vi "MGCC_StaEst_opal_RT_convertPnode.vi"(10 "cluster":T1) -> (0 "error out 2":errorcluster, 1 "error out 3":errorcluster, 2 "P_node":T1)   [LabVIEW 2016]
uses:
  Model Management/Global_MdlMgmt.vi
  <vilib>/Utility/error.llb/Error Cluster From Error Code.vi
  MGCC_StaEst_global.vi
  Finite State Machine/Sub-VIs/MGCC_FntStaMach_gobal.vi
  <vilib>/imath/engines/lvmath2/RunTimeEngine/IndexRead/NIMS M($,S).vi
  <instcachedir>/0/NIMS M($,S)_3E5749BBB62E49528D4765A77F1F6D98.lvgen/NIMS M($,S)_3E5749BBB62E49528D4765A77F1F6D98_001.vi
  <vilib>/imath/engines/lvmath2/RunTimeEngine/BuiltInFunctions/length/NIMS_length(GV).vi
  <instcachedir>/0/NIMS_length(GV)_08A3D13377FD4E4B96F5795FBF3698FA.lvgen/NIMS_length(GV)_08A3D13377FD4E4B96F5795FBF3698FA_001.vi
  <vilib>/imathl/engines/lvmath/Functions/Error Handling/Create Error.vi
  <vilib>/imath/engines/lvmath2/RunTimeEngine/RangeToken/NIMS_Range_R3 - Integer.vi
  <instcachedir>/0/NIMS_Range_R3 - Integer_A435E2FF893B4C718FD5055FE39FE2F6.lvgen/NIMS_Range_R3 - Integer_A435E2FF893B4C718FD5055FE39FE2F6_000.vi
  <vilib>/imath/engines/lvmath2/RunTimeEngine/CommandStatement/MC_CommandStatement_break.vi
  <vilib>/imath/engines/lvmath2/RunTimeEngine/IndexRead/NIMS V(S).vi
  <instcachedir>/0/NIMS V(S)_0488751826AF41519A22953C041130DC.lvgen/NIMS V(S)_0488751826AF41519A22953C041130DC_000.vi
  <vilib>/imath/engines/lvmath2/RunTimeEngine/IndexReplace/NIMS M(S,$)=V.vi
  <instcachedir>/0/NIMS M(S,$)=V_BCCFA522A894489B8FA760383D74A164.lvgen/NIMS M(S,$)=V_BCCFA522A894489B8FA760383D74A164_001.vi
  <instcachedir>/0/NIMS M($,S)_3E5749BBB62E49528D4765A77F1F6D98.lvgen/NIMS M($,S)_3E5749BBB62E49528D4765A77F1F6D98_000.vi
  <instcachedir>/0/NIMS_length(GV)_08A3D13377FD4E4B96F5795FBF3698FA.lvgen/NIMS_length(GV)_08A3D13377FD4E4B96F5795FBF3698FA_000.vi
  <vilib>/imath/engines/lvmath2/RunTimeEngine/IndexRead/NIMS M(S,S).vi
  <instcachedir>/0/NIMS M(S,S)_AC51E74150A542F7991B9634C66F3096.lvgen/NIMS M(S,S)_AC51E74150A542F7991B9634C66F3096_000.vi
  <vilib>/imath/engines/lvmath2/RunTimeSupport/NIMS_Error if Not Equal.vi
  <instcachedir>/0/NIMS_Error if Not Equal_43252A79AD05436189442EC0C5E5AB8A.lvgen/NIMS_Error if Not Equal_43252A79AD05436189442EC0C5E5AB8A_000.vi
  <vilib>/imath/engines/lvmath2/RunTimeEngine/ErrorHandling/NIMS_Create Error From Enums.vi
  <vilib>/imath/engines/lvmath2/RunTimeEngine/IndexRead/NIMS M(S,$).vi
  <instcachedir>/0/NIMS M(S,$)_F24F360562DE41D8BE234322A2E15C65.lvgen/NIMS M(S,$)_F24F360562DE41D8BE234322A2E15C65_001.vi
  <vilib>/imath/engines/lvmath2/RunTimeEngine/NodeEndStatement/NIMS_NodeEndStatement_Output.vi
  <instcachedir>/0/NIMS_NodeEndStatement_Output_53EC0D466D134D7ABD903AC30B43404B.lvgen/NIMS_NodeEndStatement_Output_53EC0D466D134D7ABD903AC30B43404B_003.vi
  <vilib>/imath/engines/lvmath2/RunTimeEngine/ErrorHandling/NIMS_Finalize Error.vi
  <vilib>/ErrorRing/Error Ring.xnode
panel:
  out "array w/ subset deleted":dbl[](array[numeric])
  out "f_MGCC_OnliTopoIden_EnergizedMatrix 2":dbl[](array[numeric])
  out "State_est BESS location":dbl[](array[numeric])
  out "Slack_bus":dbl[](array[numeric])
  out "element":dbl
  out "f_MGCC_OnliTopoIden_EnergizedMatrix":dbl[](array[numeric])
  out "error out":errorcluster
  out "p_node 2":cdb[][](array[numeric])
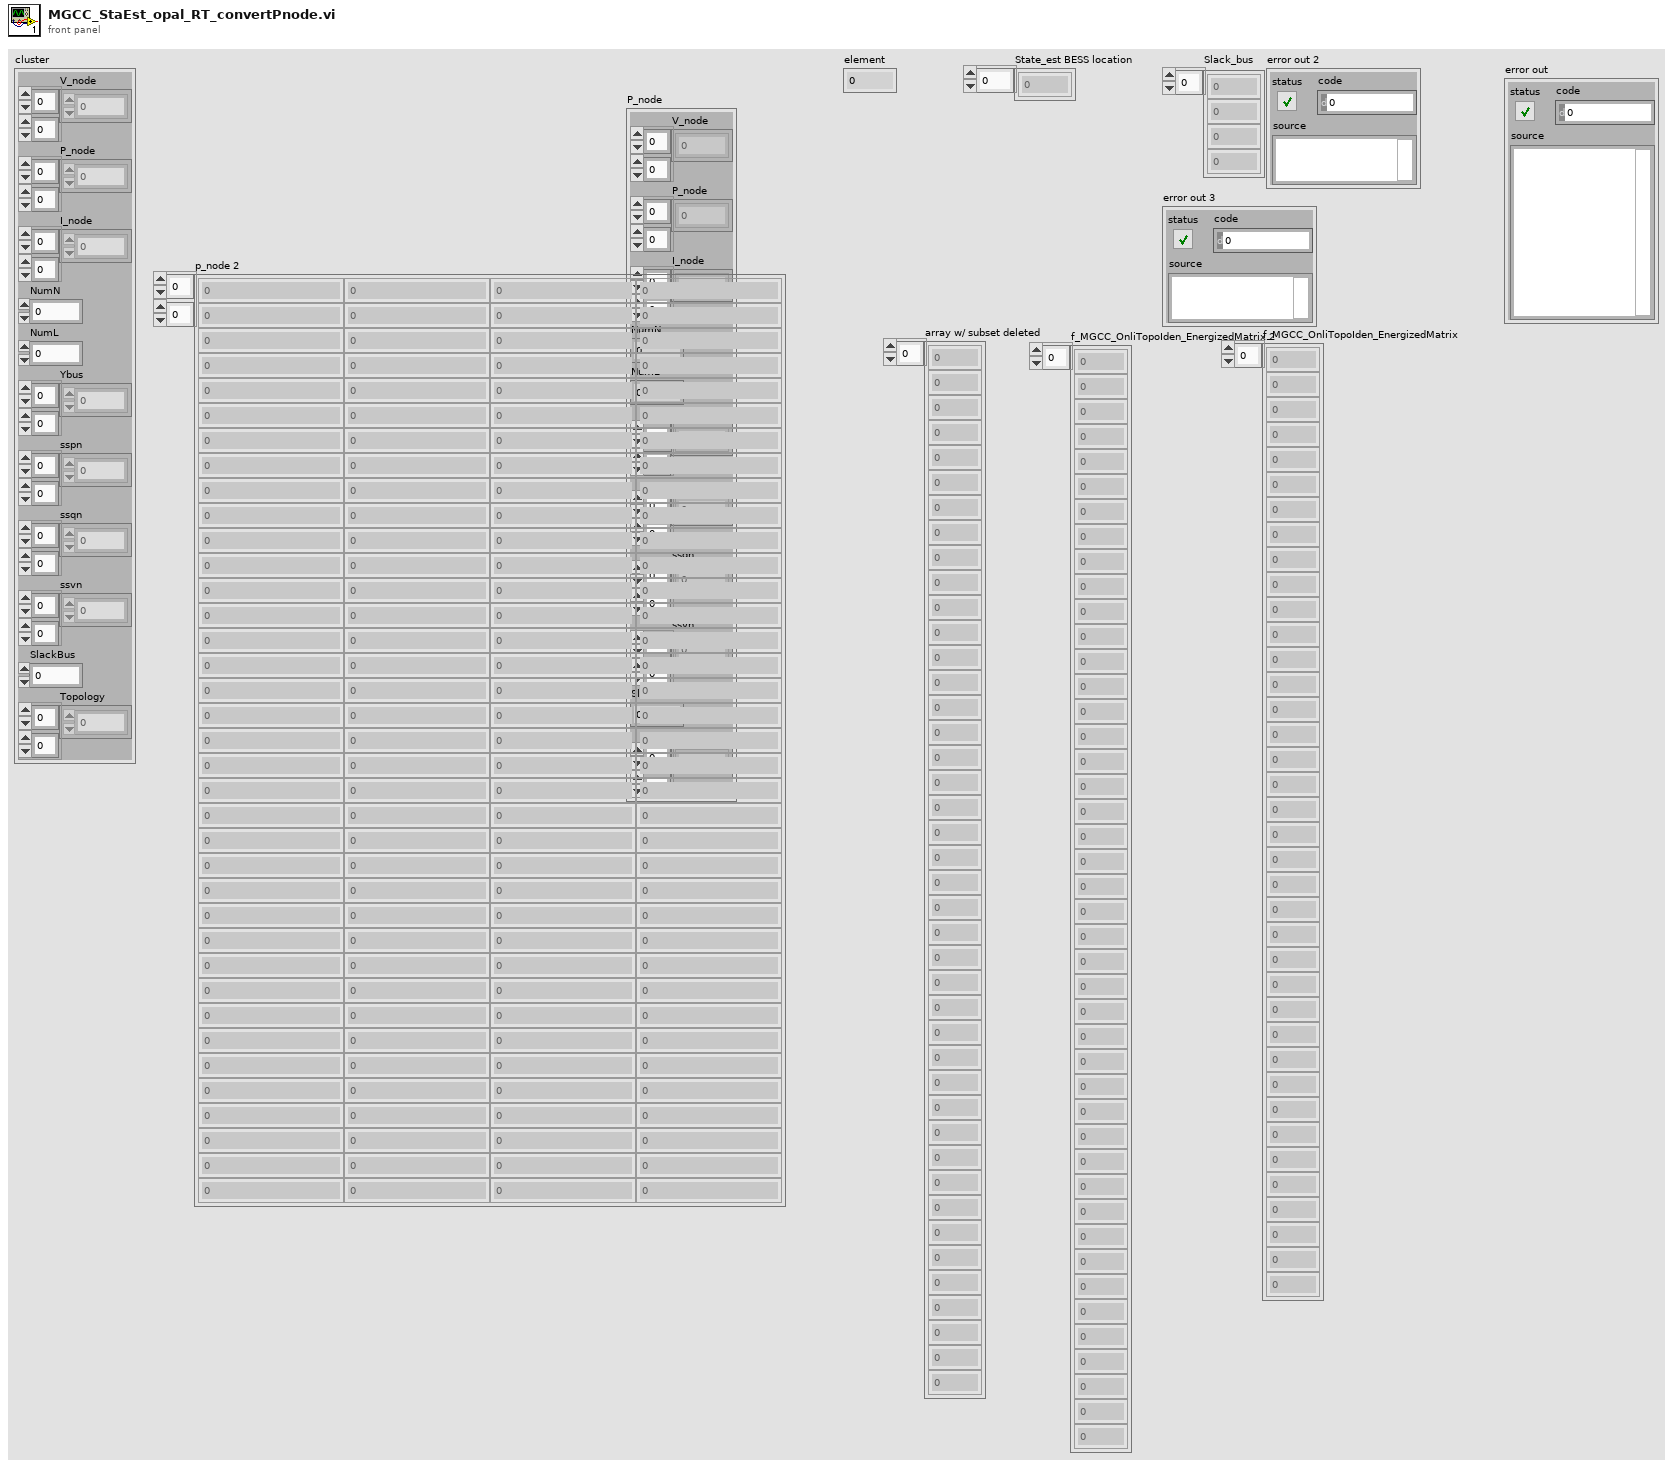
[diagram p1: front panel]
types:
  T1 = cluster{"V_node":cdb[][], "P_node":cdb[][], "I_node":cdb[][], "NumN":dbl, "NumL":dbl, "Ybus":cdb[][], "sspn":dbl[][], "ssqn":dbl[][], "ssvn":dbl[][], "SlackBus":dbl, "Topology":dbl[][]}
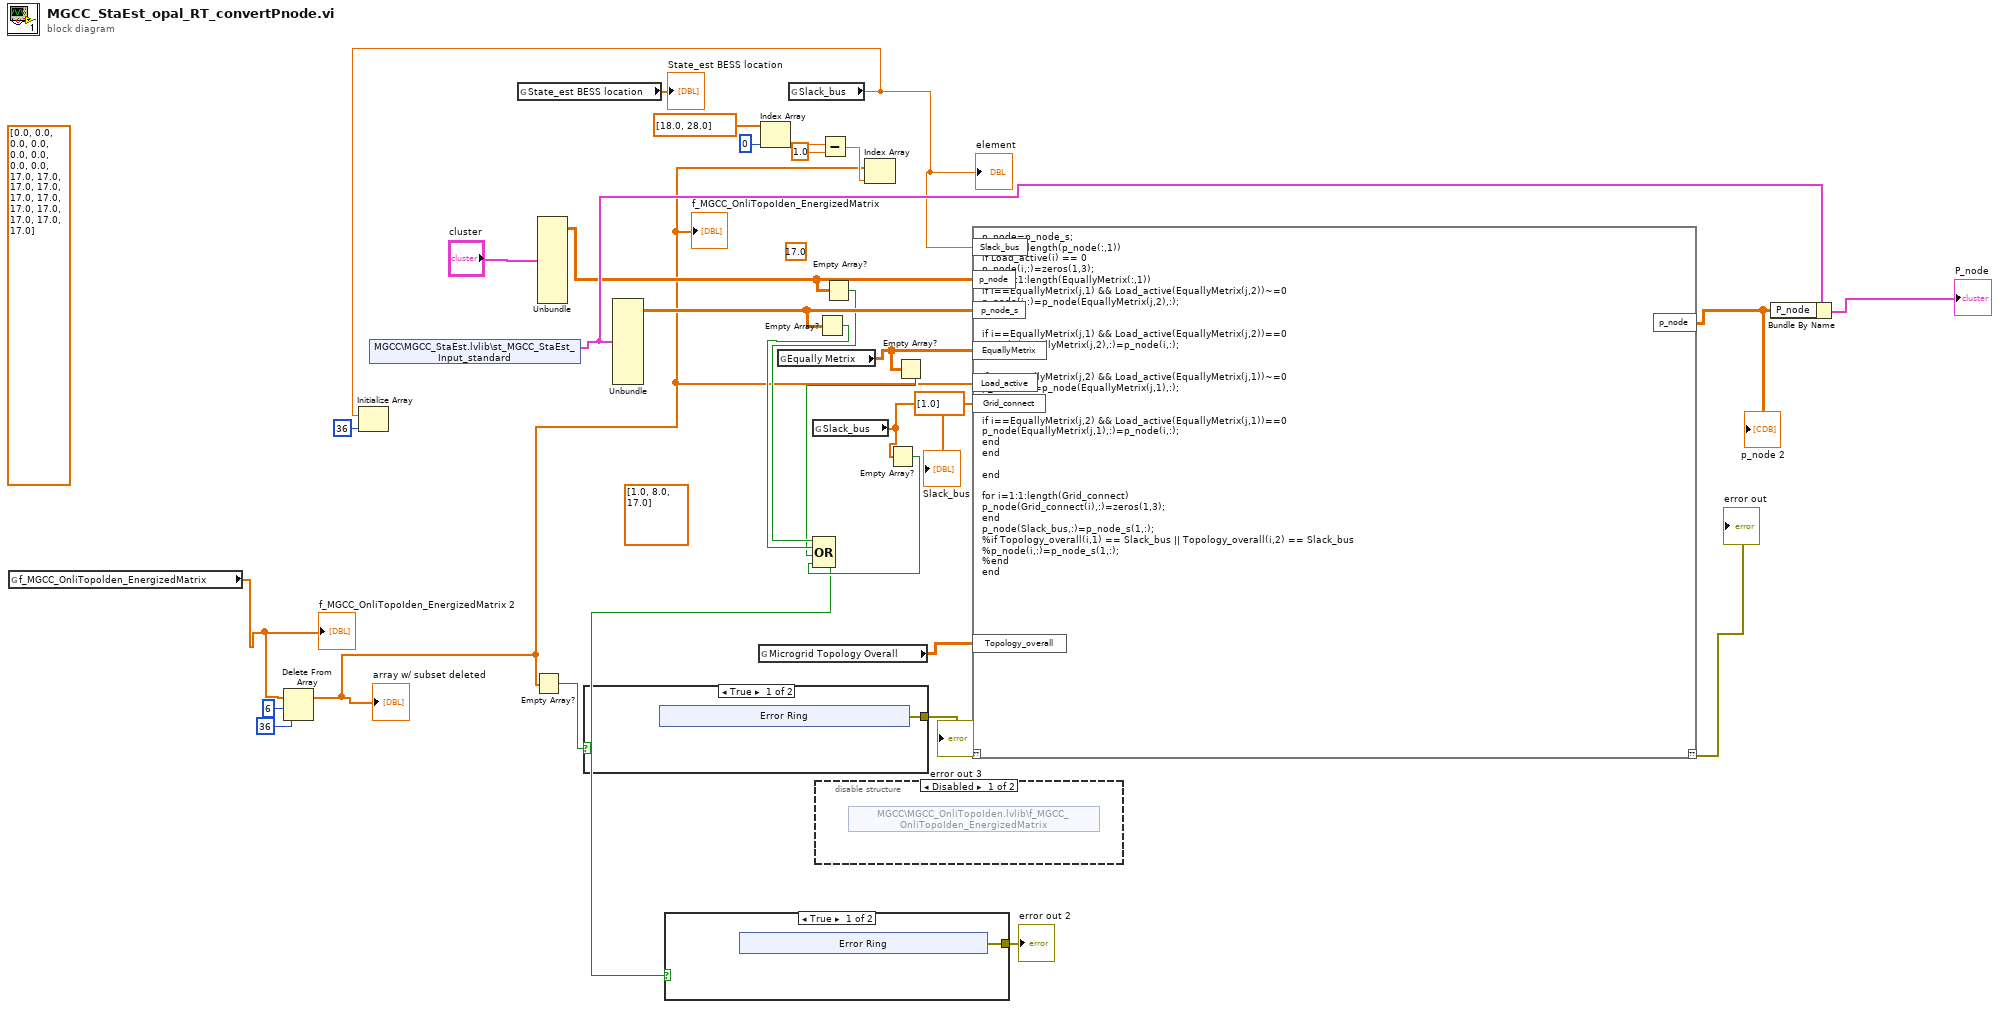
[diagram p0: block diagram]
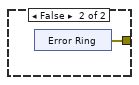
[diagram p2: hidden frame]
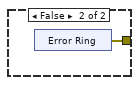
[diagram p3: hidden frame]
diagram:
  (unwired) dbl[] [0.0, 0.0, 0.0, 0.0, 0.0, 0.0, 0.0, 0.0, 17.0, 17.0, 17.0, 17.0, 17.0, 17.0, 17.0, 17.0, 17.0, 17.0, 17.0] ("Load_active")
  (unwired) dbl[] [1.0, 8.0, 17.0] ("Grid_connect")
  (unwired) 17.0 ("Slack_bus")
  n1 = global read "MGCC_FntStaMach_gobal.vi" "f_MGCC_OnliTopolden_EnergizedMatrix"() -> (w1:dbl[])
  "f_MGCC_OnliTopoIden_EnergizedMatrix 2" <- w1
  n2 = Delete From Array(array=w1, length=6, index=36) -> (array with subset deleted=w3:dbl[])  [unwired: 1 out]
  "f_MGCC_OnliTopoIden_EnergizedMatrix" <- w3
  "array w/ subset deleted" <- w3
  n3 = shared-variable "MGCC\\MGCC_StaEst.lvlib\\st_MGCC_StaEst_Input_standard"() -> (w24:T1)  [unwired: 1 in, 1 out]
  n4 = global read "Global_MdlMgmt.vi" "State_est BESS location"() -> (→"State_est BESS location":dbl[])
  n5 = Empty Array?(array=w3) -> (empty?=w12:bool)
  n6 = Unbundle("cluster") -> ("P_node"=w22:cdb[][])  [unwired: 10 out]
  n7 = case shown="True" w12 {
    tunnel: [w32 w38] -> w11
    frame True {
      n8 = xnode "Error Ring"() -> ("error out"=w32:errorcluster)
    }
    frame False {
      n9 = xnode "Error Ring"() -> ("error out"=w38:errorcluster)
    }
  }
  "error out 3" <- w11
  n10 = Unbundle(w24) -> ("P_node"=w21:cdb[][])  [unwired: 10 out]
  n11 = global read "Global_MdlMgmt.vi" "Microgrid Topology Overall"() -> (w2:dbl[][])
  n12 = Index Array(array=dbl[] [18.0, 28.0], index=0) -> (element=w27:dbl)
  n13 = global read "Global_MdlMgmt.vi" "Equally Metrix"() -> (w20:dbl[][])
  n14 = global read "MGCC_StaEst_global.vi" "Slack_bus"() -> (w6:dbl)
  "element" <- w6
  n15 = Initialize Array(w6, 36 ("dimension size")) -> ()  [unwired: 1 out]
  n16 = global read "Global_MdlMgmt.vi" "Slack_bus"() -> (w19:dbl[])
  "Slack_bus" <- w19
  n17 = disable-structure shown="Disabled" {
    frame Disabled {
      n18 = shared-variable "MGCC\\MGCC_OnliTopoIden.lvlib\\f_MGCC_OnliTopoIden_EnergizedMatrix"() -> ()  [unwired: 1 in, 2 out]
    }
    frame Enabled {
    }
  }
  n19 = Empty Array?(array=w21) -> (empty?=w17:bool)
  n20 = Subtract(x=w27, y=1.0) -> (x-y=w25:dbl)
  n21 = Empty Array?(array=w22) -> (empty?=w18:bool)
  n22 = Index Array(array=w3, index=w25) -> ()  [unwired: 1 out]
  n23 = Empty Array?(array=w19) -> (empty?=w15:bool)
  n24 = Empty Array?(array=w20) -> (empty?=w16:bool)
  n25 = Compound Arithmetic op=OR(w18, w17, w16, w15) -> (w14:bool)
  n26 = case shown="True" w14 {
    tunnel: [w40 w46] -> w13
    frame True {
      n27 = xnode "Error Ring"() -> ("error out"=w40:errorcluster)
    }
    frame False {
      n28 = xnode "Error Ring"() -> ("error out"=w46:errorcluster)
    }
  }
  "error out 2" <- w13
  n29 = mathscript code="p_node=p_node_s;\nfor i=1:1:length(p_node(:,1))\nif Load_active(i) == 0\np_node(i,:)=zeros(1,3);\nfor j=1:1:length(EquallyMetrix(:,1))\nif i==EquallyMetrix(j,1) && Load_active(EquallyMetrix(j,2))~=0\np_node(i,:)=p_node(EquallyMetrix(j,2),:);\nend\n\nif i==EquallyMetrix(j,1) && Load_active(EquallyMetrix(j,2))==0\np_node(EquallyMetrix(j,2),:)=p_node(i,:);\nend\n\nif i==EquallyMetrix(j,2) && Load_active(EquallyMetrix(j,1))~=0\np_node(i,:)=p_node(EquallyMetrix(j,1),:);\nend\n\nif i==EquallyMetrix(j,2) && Load_active(EquallyMetrix(j,1))==0\np_node(EquallyMetrix(j,1),:)=p_node(i,:);\nend\nend\n\nend\n\nfor i=1:1:length(Grid_connect)\np_node(Grid_connect(i),:)=zeros(1,3);\nend\np_node(Slack_bus,:)=p_node_s(1,:);\n%if Topology_overall(i,1) == Slack_bus || Topology_overall(i,2) == Slack_bus\n%p_node(i,:)=p_node_s(1,:);\n%end\nend"("p_node"=w22, "p_node_s"=w21, "EquallyMetrix"=w20, "Load_active"=w3, "Slack_bus"=w6, "Grid_connect"=dbl[] [1.0], "Topology_overall"=w2) -> ("??"=→"error out":errorcluster, "p_node"=w30:cdb[][])  [unwired: 1 in]
  "p_node 2" <- w30
  n30 = Bundle By Name(cluster=w24, "P_node"=w30) -> (→"P_node":T1)
